vi "Vision Research Phantom Series PhCon PhMakeAllIpVisible.vi"(5 "Error In (no error)":errorcluster) -> (19 "Error Out":errorcluster)   [LabVIEW 2013, in "VRI.lvlib"]
doc: "PhMakeAllIpVisible\nHRESULT PhMakeAllIpVisible(void)\n\nNo Parameters\n\nReturn Value\nThe function returns ERR_Ok in case of success or an error code, otherwise. To get extended error information call PhGetErrorMessage.\n\nRemarks\nEmpties both the Visible and the Ignored camera lists. This way, any camera will become visible.\n\nRequired Header\nPhCon.h"
uses:
  VRI.lvlib
  Phantom DLLs/PhCon.Dll
panel:
  # "For instructions on the use of this VI, press Ctrl+H to display the help window and move the mouse over the icon, controls, and indicators"
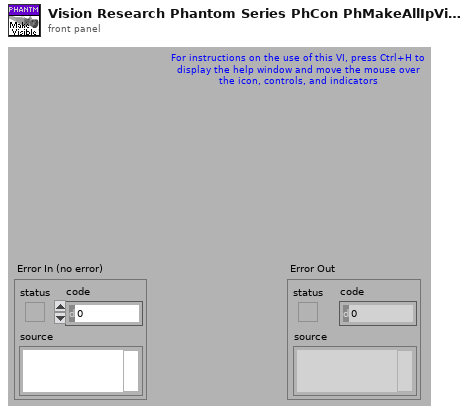
[diagram p1: front panel]
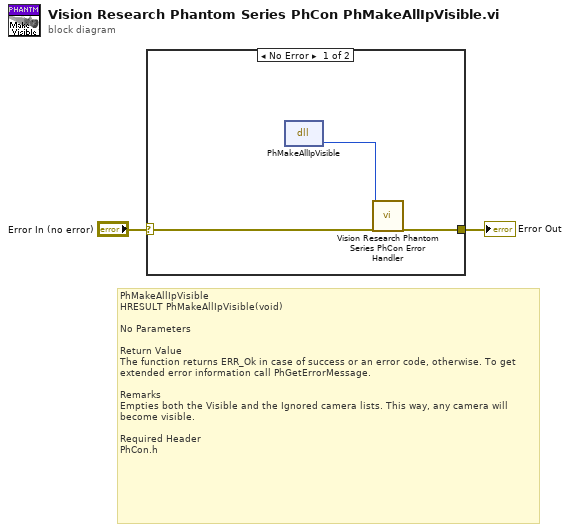
[diagram p0: block diagram]
diagram:
  # "PhMakeAllIpVisible\nHRESULT PhMakeAllIpVisible(void)\n\nNo Parameters\n\nReturn Value\nThe function returns ERR_Ok in case of success or an error code, otherwise. To get extended error information call PhGetErrorMessage.\n\nRemarks\nEmpties both the Visible and the Ignored camera lists. This way, any camera will become visible.\n\nRequired Header\nPhCon.h"
  n1 = case shown="No Error" "Error In (no error)" {
    selector: "Error In (no error)" -> [w5 w6]
    tunnel: [w4 w6] -> w1
    frame No Error {
      n2 = dll-call lib="C:/Projects/SDK/64-bit/Vision Research Phantom Series Labview Driver/Phantom DLLs/PhCon.dll" fn="PhMakeAllIpVisible"() -> ("HRESULT"=w3:i32)  [unwired: 3 in, 2 out]
      n3 = call "Vision Research Phantom Series PhCon Error Handler.vi"("ErrNo"=w3, "Error In (no error)"=w5) -> ("Error Out"=w4:errorcluster)  [unwired: 17 out]
    }
    frame Error {
    }
  }
  "Error Out" <- w1
